vi "Import Configuration.vi"(8 "error in (no error)":errorcluster, 11 "Node Ptr":u64 format="%.0x") -> (0 "error out":errorcluster)   [LabVIEW 2024, in "Embedded TDMS Logger System Explorer.lvlib"]
doc: "Allow the user to select either a CSV or XML file and import this as a configuration of the Custom Device into the System Definition. This is useful for automated tasking of the Custom Device, CSV is legacy code but useful for non-code based users to use tools like Excel to define channels and logging groups."
uses:
  Embedded TDMS Logger System Explorer.lvlib
  <userlib>/_OpenG.lib/file/file.llb/Strip Path Extension - Path__ogtk.vi
  Shared/Constants.vi
  <vilib>/Utility/error.llb/Error Cluster From Error Code.vi
  <vilib>/ErrorRing/Error Ring.xnode
  <userlib>/_OpenG.lib/file/file.llb/openg_file.lvlib
  <vilib>/NI VeriStand/Custom Device API/Custom Device API.lvlib
  Shared/Embedded TDMS Logger Shared.lvlib
panel:
  in  "Tag":string
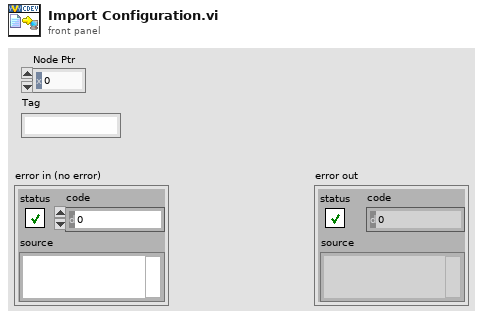
[diagram p1: front panel]
types:
  T1 = typedef "Custom Device API.lvlib/Custom Device Item Ref.ctl" = u64
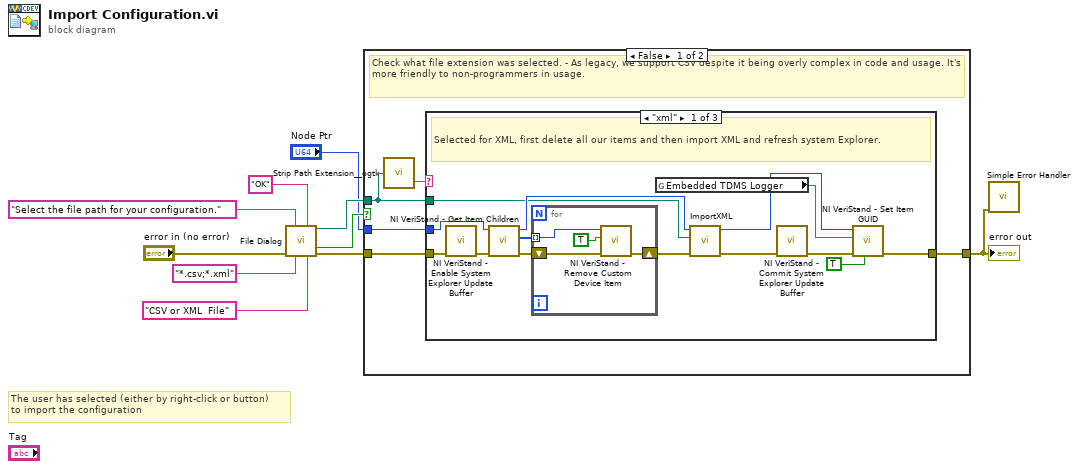
[diagram p0: block diagram]
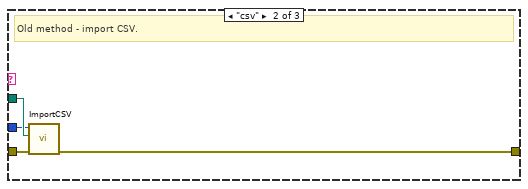
[diagram p2: hidden frame]
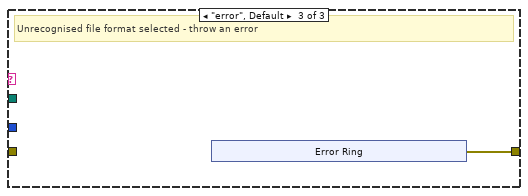
[diagram p3: hidden frame]
diagram:
  # "The user has selected (either by right-click or button)\nto import the configuration"
  n1 = call "File Dialog"("prompt"="Select the file path for your configuration.", "button label"="OK", "error in"="error in (no error)", "pattern (all files)"="*.csv;*.xml", "pattern label"="CSV or XML  File") -> ("selected path"=w8:path, "cancelled"=w10:bool, "error out"=w9:errorcluster)  [unwired: 7 in, 1 out]
  n2 = case shown="False" w10 {
    tunnel: w9 -> [w15 w44]
    tunnel: [w12 w44] -> w1
    tunnel: w8 -> [w14 _]
    tunnel: "Node Ptr" -> [w11 _]
    frame False {
      # "Check what file extension was selected. - As legacy, we support CSV despite it being overly complex in code and usage. It's more friendly to non-programmers in usage."
      n3 = call-poly <userlib>:"Strip Path Extension__ogtk.vi"("path"=w14) -> ("extension"=w13:string)  [unwired: 1 out]
      n4 = case shown="\"xml\"" w13 {
        tunnel: w15 -> [w25 w37 _]
        tunnel: w14 -> [w22 w36 _]
        tunnel: [w19 w35 w38] -> w12
        tunnel: w11 -> [w23 w34 _]
        frame "xml" {
          # "Selected for XML, first delete all our items and then import XML and refresh system Explorer."
          n5 = call <vilib>:"NI VeriStand - Enable System Explorer Update Buffer.vi"("error in (no error)"=w25) -> ("error out"=w24:errorcluster)  [unwired: 10 in]
          n6 = call <vilib>:"NI VeriStand - Get Item Children.vi"("error in (no error)"=w24, "Item Ref in"=w23) -> ("error out"=w29:errorcluster, "Child Refs"=w28:T1[], "Item Ref out"=w26:T1)  [unwired: 6 in, 1 out]
          n7 = for {
            shift-right: [w33] -> w27
            shift-left: w29 -> [w32]
            tunnel: w28 -> [w31] mode=indexing
            n8 = call <vilib>:"NI VeriStand - Remove Custom Device Item.vi"("error in (no error)"=w32, "Force Delete (F)"=TRUE, "Item Ref in"=w31) -> ("error out"=w33:errorcluster)  [unwired: 7 in, 1 out]
          }
          n9 = global read "Constants.vi" "Embedded TDMS Logger"() -> (w16:string)
          n10 = call "ImportXML.vi"("error in (no error)"=w27, "selected path"=w22, "Node Ptr"=w26) -> ("error out"=w21:errorcluster, "Node Ptr Out"=w17:T1)  [unwired: 7 in]
          n11 = call <vilib>:"NI VeriStand - Commit System Explorer Update Buffer.vi"("error in (no error)"=w21) -> ("error out"=w20:errorcluster)  [unwired: 10 in]
          n12 = call <vilib>:"NI VeriStand - Set Item GUID.vi"("Refresh System Explorer Tree? (F)"=TRUE, "error in (no error)"=w20, "GUID"=w16, "Item Ref in"=w17) -> ("error out"=w19:errorcluster)  [unwired: 6 in, 1 out]
        }
        frame "csv" {
          # "Old method - import CSV."
          n13 = call "ImportCSV.vi"("error in (no error)"=w37, "selected path"=w36, "Node Ref In"=w34) -> ("error out"=w35:errorcluster)  [unwired: 8 in]
        }
        frame "error", Default {
          # "Unrecognised file format selected - throw an error"
          n14 = xnode "Error Ring"() -> ("error out"=w38:errorcluster)
        }
      }
    }
    frame True {
      # "User cancelled the operation - do nothing"
    }
  }
  "error out" <- w1
  n15 = call <vilib>:"Simple Error Handler.vi"("error in (no error)"=w1) -> ()  [unwired: 4 in, 5 out]
